vi "W&R_ARDUINO2LABVIEW_1BYTE.vi"() -> ()   [LabVIEW 2019]
uses:
  <vilib>/Instr/_visa.llb/Select Event Type.ctl
  <vilib>/Instr/_visa.llb/VISA Configure Serial Port (Instr).vi
panel:
  out "event":refnum<visa-resource-name>
  out "read buffer":string
  out "x .or. y?":bool
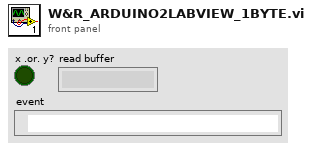
[diagram p1: front panel]
types:
  T1 = typedef "Select Event Type.ctl" = u32
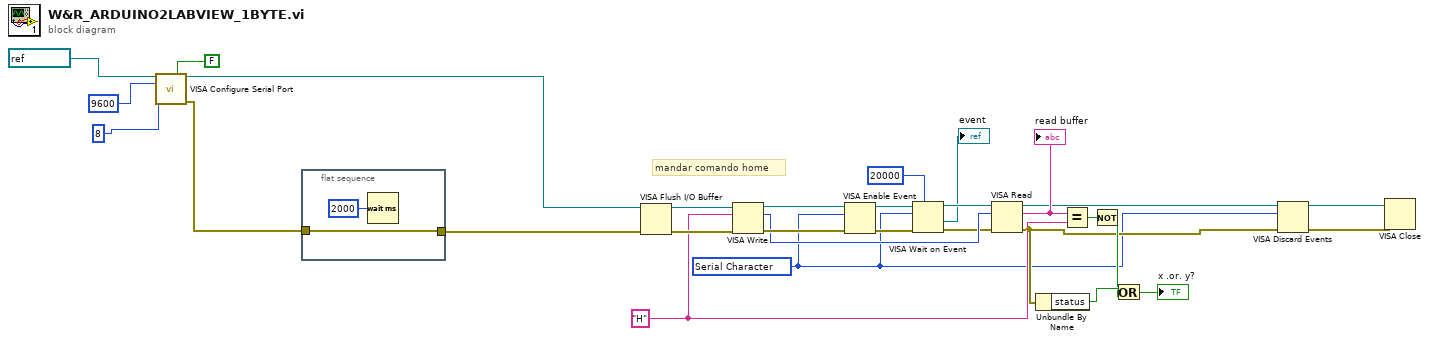
[diagram p0: block diagram]
diagram:
  w1 = T1 1073684533 items=["Service Request"=1073684491, "Trigger"=3221168138, "Clear"=1073684493, "VXI Signal"=1073684512, "VXI/VME Interrupt"=3221168161, "VXI/VME Sysfail"=1073684509, "VXI/VME Sysreset"=1073684510, "GPIB CIC"=1073684498, "GPIB Talk"=1073684499, "GPIB Listen"=1073684500, "PXI Interrupt"=1073684514, "Serial Break"=1073684515, "Serial TermChar"=1073684516, "Serial CTS"=1073684521, "Serial DSR"=1073684522, "Serial DCD"=1073684524, "Serial RI"=1073684526, "Serial Character"=1073684533, "USB Interrupt"=1073684535, "All Enabled"=1073709055] ("Event Type")
  w15 = "H" ("write buffer")
  # "mandar comando home"
  n1 = call-poly "VISA Configure Serial Port"("VISA resource name"=refnum<visa-resource-name> "COM5", "Enable Termination\nChar (T)"=FALSE ("Enable Termination\nChar (T)"), "baud rate (9600)"=u32 9600, "data bits (8)"=u16 8) -> ("VISA resource name out"=w8:refnum<visa-resource-name>, "error out"=w27:errorcluster)  [unwired: 10 in]
  n2 = flat-sequence {
    tunnel: [w31] -> w9
    tunnel: w27 -> [w31]
    frame #0 {
      n3 = Wait (ms)(milliseconds to wait=u32 2000) -> ()  [unwired: 1 out]
    }
  }
  n4 = VISA Flush I/O Buffer(VISA resource name=w8, error in (no error)=w9) -> (VISA resource name out=w24:refnum<visa-resource-name>, error out=w23:errorcluster)  [unwired: 1 in]
  n5 = VISA Write(VISA resource name=w24, write buffer=w15, error in (no error)=w23) -> (VISA resource name out=w22:refnum<visa-resource-name>, return count=w16:u32, error out=w21:errorcluster)
  n6 = VISA Enable Event(8:w21, 10:w1, 11:w22) -> (0:w19:errorcluster, 3:w20:refnum<visa-resource-name>)  [unwired: 1 in]
  n7 = VISA Wait on Event(7:u32 20000 ("timeout (0)"), 8:w19, 10:w1, 11:w20) -> (0:w13:errorcluster, 1:→"event":refnum<visa-resource-name>, 3:w17:refnum<visa-resource-name>)  [unwired: 1 in, 1 out]
  n8 = VISA Read(VISA resource name=w17, byte count=w16, error in (no error)=w13) -> (VISA resource name out=w5:refnum<visa-resource-name>, read buffer=w14:string, error out=w4:errorcluster)  [unwired: 1 out]
  "read buffer" <- w14
  n9 = Unbundle By Name(w4) -> ("status"=w12:bool)
  n10 = Equal?(x=w14, y=w15) -> (x = y?=w11:bool)
  n11 = Not(x=w11) -> (.not. x?=w10:bool)
  n12 = Or(x=w12, y=w10) -> (x .or. y?=→"x .or. y?":bool)
  n13 = VISA Discard Events(8:w4, 10:w1, 11:w5) -> (0:w2:errorcluster, 3:w3:refnum<visa-resource-name>)  [unwired: 1 in]
  n14 = VISA Close(VISA resource name=w3, error in (no error)=w2) -> ()  [unwired: 1 out]
